vi "Load Deployment Hooks.vi"(8 "error in":errorcluster) -> (0 "error out":errorcluster, 3 "iCDDepHooks out":refnum<class "CustomDeviceDeploymentHooks.lvclass">)   [LabVIEW 2026, in "Template Configuration.lvlib"]
uses:
  Template Configuration.lvlib
  <vilib>/Utility/LVLibp/NI_PackedLibraryUtility.lvlib
  <vilib>/Utility/error.llb/whitespace.ctl
  <vilib>/Utility/error.llb/Trim Whitespace (string).vi
  <userlib>/CustomDeviceInterfaces_v1.lvlibp/custom-device-express-framework/Source/Custom Device Interfaces/CustomDeviceDeploymentHooks/CustomDeviceDeploymentHooks.lvclass
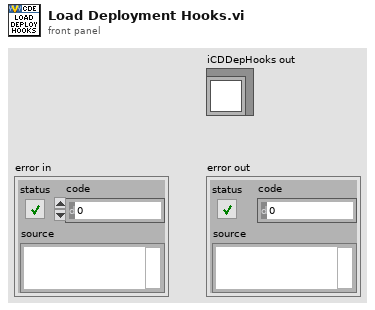
[diagram p1: front panel]
types:
  T1 = typedef "whitespace.ctl" = u16
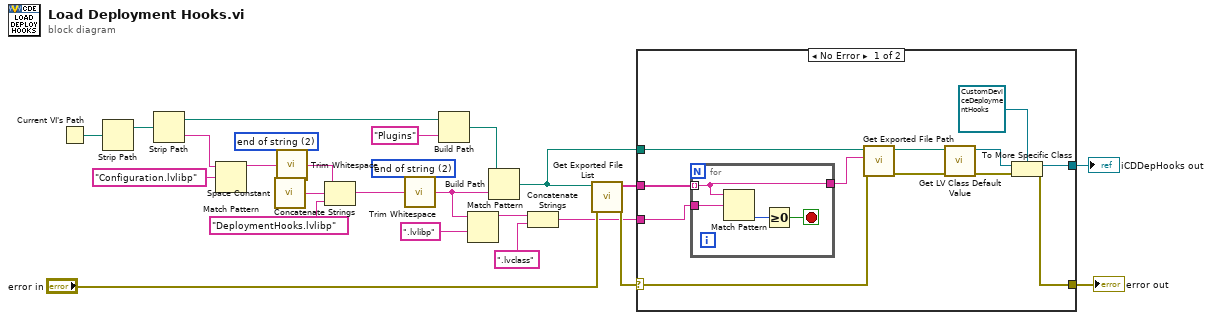
[diagram p0: block diagram]
diagram:
  w6 = T1 2 items=["both", "start of string", "end of string"] ("location (both)")
  w10 = T1 2 items=["both", "start of string", "end of string"] ("location (both)")
  n1 = Current VI's Path() -> (path=w1:path)
  n2 = Strip Path(path=w1) -> (stripped path=w17:path)  [unwired: 1 out]
  n3 = Strip Path(path=w17) -> (stripped path=w13:path, name=w15:string)
  n4 = Match Pattern(string=w15, regular expression="Configuration.lvlibp") -> (before substring=w5:string)  [unwired: 1 in, 3 out]
  n5 = call <vilib>:"Space Constant.vi"() -> ("String"=w11:string)
  n6 = call-poly <vilib>:"Trim Whitespace.vi"("string"=w5, "location (both)"=w6) -> ("trimmed string"=w7:string)
  n7 = Concatenate Strings(w7, w11, "DeploymentHooks.lvlibp") -> (w8:string)
  n8 = call-poly <vilib>:"Trim Whitespace.vi"("string"=w8, "location (both)"=w10) -> ("trimmed string"=w4:string)
  n9 = Build Path(base path=w13, name or relative path="Plugins") -> (appended path=w9:path)
  n10 = Match Pattern(string=w4, regular expression=".lvlibp") -> (before substring=w20:string)  [unwired: 1 in, 3 out]
  n11 = Build Path(base path=w9, name or relative path=w4) -> (appended path=w3:path)
  n12 = Concatenate Strings(w20, ".lvclass" ("regular expression")) -> (w18:string)
  n13 = call <vilib>:"Get Exported File List.vi"("error in (no error)"="error in", "packed library path"=w3) -> ("error out"=w23:errorcluster, "qualified names"=w22:string[])  [unwired: 7 in, 1 out]
  n14 = case shown="No Error" w23 {
    selector: w23 -> [w37 w42]
    tunnel: w22 -> [w33 _]
    tunnel: w3 -> [w32 _]
    tunnel: [w30 _] -> w2
    tunnel: [w36 w42] -> w24
    tunnel: w18 -> [w28 _]
    frame No Error {
      n15 = for {
        tunnel: w33 -> [w38] mode=indexing
        tunnel: w28 -> [w41]
        tunnel: [w38] -> w31
        stop <- w39 stop-if-true
        n16 = Match Pattern(string=w38, regular expression=w41) -> (offset past match=w40:i32)  [unwired: 1 in, 3 out]
        n17 = Greater Or Equal To 0?(x=w40) -> (x >= 0?=w39:bool)
      }
      n18 = call <vilib>:"Get Exported File Path.vi"("error in (no error)"=w37, "qualified name"=w31, "packed library path"=w32) -> ("error out"=w35:errorcluster, "path"=w27:path)  [unwired: 7 in]
      n19 = call <vilib>:"Get LV Class Default Value.vi"("error in (no error)"=w35, "class path"=w27) -> ("error out"=w34:errorcluster, "object"=w29:refnum<class>)  [unwired: 8 in]
      n20 = To More Specific Class(target class=refnum<class "CustomDeviceDeploymentHooks.lvclass"> refnum ("iPluginSettingsCompiler.lvclass"), reference=w29, error in=w34) -> (specific class reference=w30:refnum<class "CustomDeviceDeploymentHooks.lvclass">, error out=w36:errorcluster)
    }
    frame Error {
    }
  }
  "error out" <- w24
  "iCDDepHooks out" <- w2
